vi "Get Nested Child Section Node Types.vi"(8 "error in":errorcluster, 11 "Node":refnum<k20>) -> (0 "error out":errorcluster, 2 "Nested Section Types":cluster{"Nested Section Types":string[]}, 3 "Node":refnum<k20>)   [LabVIEW 2026, in "Plugin XML Parser.lvlib"]
uses:
  Plugin XML Parser.lvlib
  <vilib>/xml/Close Reference(Node).vi
  <resource>/objmgr/DOMUserDefRef.rc
  <vilib>/xml/NI_XML.lvlib
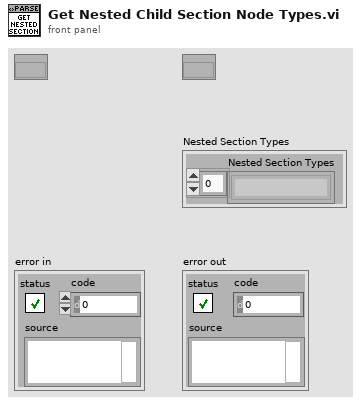
[diagram p1: front panel]
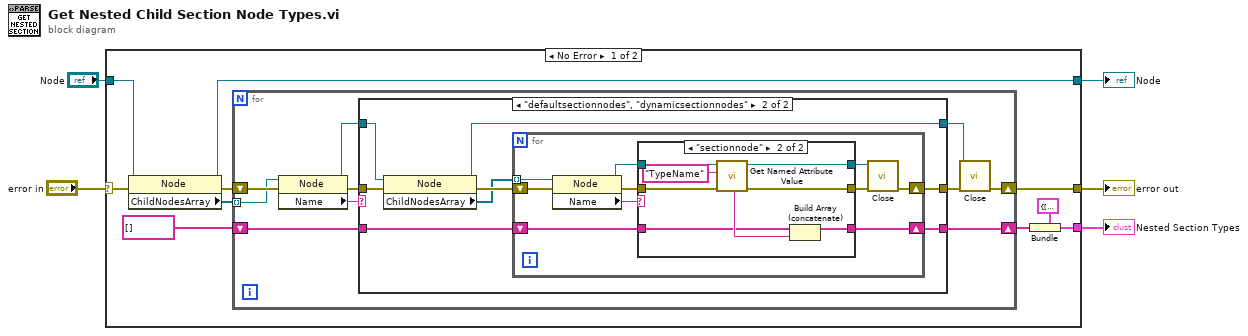
[diagram p0: block diagram]
diagram:
  n1 = case shown="No Error" "error in" {
    selector: "error in" -> [w15 w59]
    tunnel: "Node" -> [w11 w58]
    tunnel: [w13 w59] -> w4
    tunnel: [w6 _] -> w1
    tunnel: [w10 w58] -> w2
    frame No Error {
      n2 = property class="Node"(reference=w11, error in=w15) -> (reference out=w10:refnum<k20>, error out=w14:errorcluster, "ChildNodesArray"=w12:refnum<k20>[])
      n3 = for {
        tunnel: w12 -> [w21] mode=indexing
        shift-right: [w22] -> w13
        shift-left: w14 -> [w25]
        shift-right: [w17] -> w7
        shift-left: string[] [] -> [w16]
        n4 = property class="Node"(reference=w21, error in=w25) -> (reference out=w19:refnum<k20>, error out=w24:errorcluster, "Name"=w20:string)
        n5 = case shown="\"defaultsectionnodes\", \"dynamicsectionnodes\"" w20 {
          tunnel: w19 -> [w27 w33]
          tunnel: w24 -> [w28 w36]
          tunnel: [w28 w34] -> w23
          tunnel: [w26 w29] -> w17
          tunnel: [w27 w31] -> w18
          tunnel: w16 -> [w26 w30]
          frame Default {
          }
          frame "defaultsectionnodes", "dynamicsectionnodes" {
            n6 = property class="Node"(reference=w33, error in=w36) -> (reference out=w31:refnum<k20>, error out=w35:errorcluster, "ChildNodesArray"=w32:refnum<k20>[])
            n7 = for {
              tunnel: w32 -> [w42] mode=indexing
              shift-right: [w43] -> w34
              shift-left: w35 -> [w46]
              shift-right: [w37] -> w29
              shift-left: w30 -> [w38]
              n8 = property class="Node"(reference=w42, error in=w46) -> (reference out=w40:refnum<k20>, error out=w45:errorcluster, "Name"=w41:string)
              n9 = case shown="\"sectionnode\"" w41 {
                tunnel: w40 -> [w48 w55]
                tunnel: w45 -> [w49 w57]
                tunnel: [w49 w56] -> w44
                tunnel: [w48 w54] -> w39
                tunnel: [w47 w52] -> w37
                tunnel: w38 -> [w47 w51]
                frame Default {
                }
                frame "sectionnode" {
                  n10 = call "Get Named Attribute Value.vi"("error in"=w57, "Attribute Name"="TypeName", "Node In"=w55) -> ("error out"=w56:errorcluster, "Node Out"=w54:refnum<k20>, "Attribute Value"=w53:string)  [unwired: 5 in, 1 out]
                  n11 = Build Array (concatenate)(w51, w53) -> (w52:string[])
                }
              }
              n12 = call-poly <vilib>:"Close.vi"("error in (no error)"=w44, "node"=w39) -> ("error out"=w43:errorcluster)  [unwired: 7 in]
            }
          }
        }
        n13 = call-poly <vilib>:"Close.vi"("error in (no error)"=w23, "node"=w18) -> ("error out"=w22:errorcluster)  [unwired: 7 in]
      }
      n14 = Bundle(cluster=cluster{"Nested Section Types 2":string[]} {"Nested Section Types 2"=["SectionP1", "SectionQ1", "SectionR1"]} ("Nested Section Types 2"), "Nested Section Types 2"=w7) -> (w6:cluster{"Nested Section Types 2":string[]})
    }
    frame Error {
    }
  }
  "error out" <- w4
  "Node" <- w2
  "Nested Section Types" <- w1
